vi "artificial_XYZ_Motor.vi"() -> ()   [LabVIEW 2012]
panel:
  in  "Add Z Position":bool
  in  "Set Z Position":bool
  in  "stop":bool
  in  "posZ":dbl
  # "Artificial XYZ Motor"
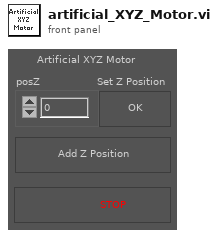
[diagram p1: front panel]
types:
  T1 = cluster{"moveXabs":dbl, "moveYabs":dbl, "moveZabs":dbl}
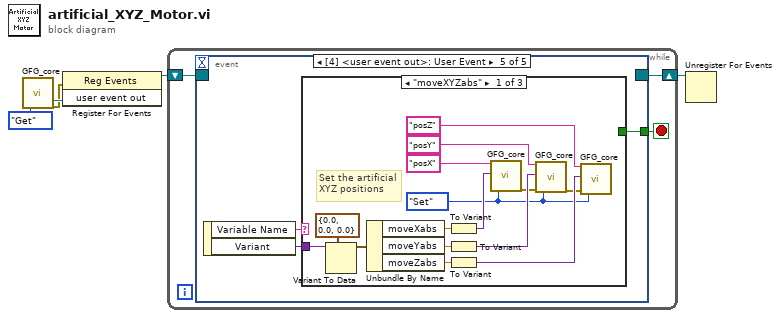
[diagram p0: block diagram]
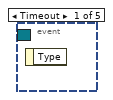
[diagram p2: hidden frame]
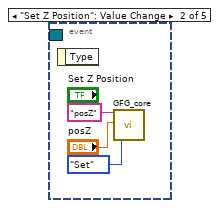
[diagram p3: hidden frame]
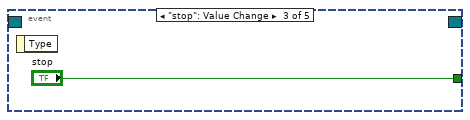
[diagram p4: hidden frame]
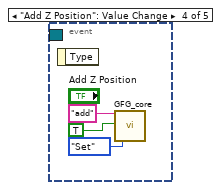
[diagram p5: hidden frame]
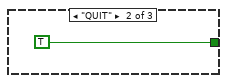
[diagram p6: hidden frame]
diagram:
  n1 = call "GFG_core.vi"("Action"=enum16{"Init", "Set", "Get", "Clear"}."Get") -> ("user event out"=w5:refnum<user-event>, "error out"=w2:errorcluster)  [unwired: 12 in, 5 out]
  n2 = register-events(error in=w2, w5) -> (reference out=w4:refnum<event-registration>)  [unwired: 1 in, 1 out]
  n3 = while {
    shift-right: [w6] -> w1
    shift-left: w4 -> [w7]
    stop <- w8 stop-if-true
    n4 = event shown="[4] <user event out>: User Event" {
      selector: w7 -> [_ _ _ _ _]
      dyn-events: [_ _ _ _ _] -> w6
      timeout: _ -> [_ _ _ _ _]
      tunnel: [_ _ "stop" _ w16] -> w8
      event Timeout {
        n5 = event-data() -> ()  [unwired: 1 in, 1 out]
      }
      event "Set Z Position": Value Change {
        n6 = event-data() -> ()  [unwired: 1 in, 1 out]
        n7 = call "GFG_core.vi"("Variable Name in"="posZ", "Variant in"="posZ", "Action"=enum16{"Init", "Set", "Get"}."Set") -> ()  [unwired: 10 in, 7 out]
      }
      event "stop": Value Change {
        n8 = event-data() -> ()  [unwired: 1 in, 1 out]
      }
      event "Add Z Position": Value Change {
        n9 = event-data() -> ()  [unwired: 1 in, 1 out]
        n10 = call "GFG_core.vi"("Variable Name in"="add", "Variant in"=TRUE, "Action"=enum16{"Init", "Set", "Get"}."Set") -> ()  [unwired: 10 in, 7 out]
      }
      event User Event {
        n11 = event-data() -> ("Variable Name"=w17:string, "Variant"=w18:variant)  [unwired: 1 in]
        n12 = case shown="\"moveXYZabs\"" w17 {
          tunnel: w18 -> [w20 _ _]
          tunnel: [_ TRUE _] -> w16
          frame "moveXYZabs" {
            w19 = enum16{"Init", "Set", "Get", "Clear"}."Set" ("Action")
            # "Set the artificial\nXYZ positions"
            n13 = Variant To Data(type=T1 {"moveXabs"=0.0, "moveYabs"=0.0, "moveZabs"=0.0} ("output cluster"), Variant=w20) -> (data=w25:T1)  [unwired: 1 in, 1 out]
            n14 = Unbundle By Name(w25) -> ("moveXabs"=w28:dbl, "moveYabs"=w29:dbl, "moveZabs"=w30:dbl)
            n15 = To Variant(anything=w28) -> (Variant=w31:variant)
            n16 = To Variant(anything=w29) -> (Variant=w32:variant)
            n17 = To Variant(anything=w30) -> (Variant=w33:variant)
            n18 = call "GFG_core.vi"("Variable Name in"="posX", "Variant in"=w31, "Action"=w19) -> ("error out"=w27:errorcluster)  [unwired: 10 in, 6 out]
            n19 = call "GFG_core.vi"("Variable Name in"="posY", "Variant in"=w32, "error in (no error)"=w27, "Action"=w19) -> ("error out"=w26:errorcluster)  [unwired: 9 in, 6 out]
            n20 = call "GFG_core.vi"("Variable Name in"="posZ", "Variant in"=w33, "error in (no error)"=w26, "Action"=w19) -> ()  [unwired: 9 in, 7 out]
          }
          frame "QUIT" {
          }
          frame Default {
          }
        }
      }
    }
  }
  n21 = Unregister For Events(event registration refnum=w1) -> ()  [unwired: 1 in, 1 out]
